vi "Configure Measurement (Edge Time).vi"(5 "Upper Percent  (90 Percent)":dbl=90.0 format="%#_4g", 7 "Lower Percent  (10 Percent)":dbl=10.0 format="%#_4g", 8 "error in (no error)":errorcluster, 9 "Edge Time Type (0:Rise)":i32(ring) items=["Rise", "Fall"], 10 "Channel (1:Channel 1)":i32(ring)=1 items=["Channel 1"=1, "Channel 2"=2], 11 "VISA resource name":refnum<visa-resource-name>) -> (0 "error out":errorcluster, 3 "VISA resource name out":refnum<visa-resource-name>)   [LabVIEW 2024, in "Agilent 532XX Series.lvlib"]
doc: "Configures the settings required for Edge Time measurements.\n\n<B>Note:</B> This VI only applies to the Agilent 53220A/53230A."
uses:
  Agilent 532XX Series.lvlib
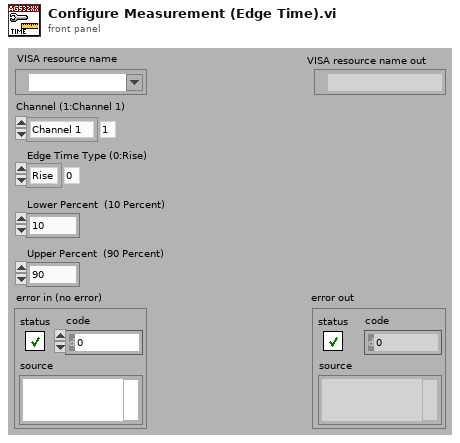
[diagram p1: front panel]
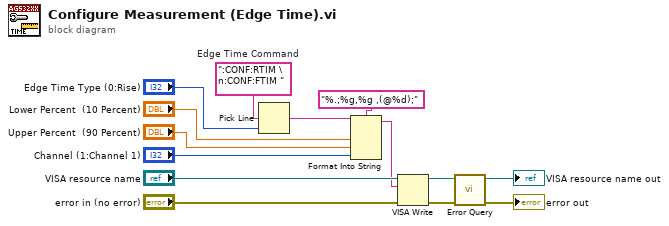
[diagram p0: block diagram]
diagram:
  w8 = ":CONF:RTIM \n:CONF:FTIM "  # Edge Time Command
  n1 = Pick Line(multi-line string=w8, line index="Edge Time Type (0:Rise)") -> (output string=w3:string)  [unwired: 1 out]
  n2 = Format Into String(format string="%.;%g,%g ,(@%d);", initial string=w3, "Lower Percent  (10 Percent)", "Upper Percent  (90 Percent)", "Channel (1:Channel 1)") -> (resulting string=w1:string)  [unwired: 1 in, 1 out]
  n3 = VISA Write(VISA resource name="VISA resource name", write buffer=w1, error in (no error)="error in (no error)") -> (VISA resource name out=w12:refnum<visa-resource-name>, error out=w10:errorcluster)  [unwired: 1 out]
  n4 = call "Error Query.vi"("error in (no error)"=w10, "VISA resource name"=w12) -> ("error out"=→"error out":errorcluster, "VISA resource name out"=→"VISA resource name out":refnum<visa-resource-name>)  [unwired: 8 out]
